vi "Actor Core.vi"(8 "error in":errorcluster, 11 "Lockin Processor in":refnum<class "Lockin Processor.lvclass">) -> (0 "error out":errorcluster, 3 "Actor out":refnum<class "Actor.lvclass">)   [LabVIEW 2016, in "Lockin Processor.lvclass"]
doc: "(<B>Filename</B>: Actor Framework.lvlib:Actor.lvclass:Actor Core.vi)\n\nReceives messages to the actor, reacts to them, and initiates any error handling that may shut the actor down.\n\nDescendant classes may override this VI to append parallel tasks for the actor to complete while it handles messages. Overrides use the Call Parent Method node."
uses:
  Lockin Processor.lvclass
  C:/github/LabActor/Template Module/Template Module.lvclass
  C:/Program Files/National Instruments/LabVIEW 2016/vi.lib/ActorFramework/Actor/Actor.lvclass
  <vilib>/ActorFramework/Actor/Actor.lvclass
  Lockin Processor Configuration.ctl
  Lockin Processor.lvclass/Lockin Processor.ctl
  Template Module/Template Module.lvclass/Template Module.ctl
  <vilib>/ActorFramework/Actor/Actor.lvclass/Actor.ctl
  <vilib>/ActorFramework/Message Enqueuer/Message Enqueuer.lvclass/Message Enqueuer.ctl
  NHMFL_Core/Libraries/Instruments/Results/File Path Result/File Path Result.lvclass
  C:/github/NHMFL_Core/Libraries/Instruments/Results/Acquired Result/Acquired Result.lvclass
  Process Object Messages/Process Result Msg/Process Result Msg.lvclass/Process Result Msg.ctl
  Template Module/Read stop event.vi
  <vilib>/ActorFramework/Message Enqueuer/Init from Existing Queue.vi
  <vilib>/ActorFramework/Message Enqueuer/Enqueue.vi
  Process Object Messages/Process Result Msg/Process Result Msg.lvclass
  C:/Program Files/National Instruments/LabVIEW 2016/vi.lib/ActorFramework/Message/Message.lvclass
  Lockin Processor Messages/Update Plot Msg/Update Plot Msg.lvclass
  <vilib>/ActorFramework/Message Priority Queue/Priority Enqueue.vi
  Process Object/Process Object.lvclass
  <vilib>/ActorFramework/Message Enqueuer/Message Enqueuer.lvclass
panel:
  out "Name":string
  in  "Re-process":bool
  out "XY Graph":cluster{dbl[], "Y":dbl[]}[](graph)
  in  "Input file":path
  in  "Configuration":T1={"Time constant"=0.0001, "Signal channels"=["V"], "Group"="p", "X channel"="Field", "Live update"=TRUE, "Phases"=[], "Harmonics"=[]} {"Phases" scale=-180.0..180.0; "Time constant" min=1e-06 max=1.0 scale=1e-06..0.01 scale format="%#_6p"}
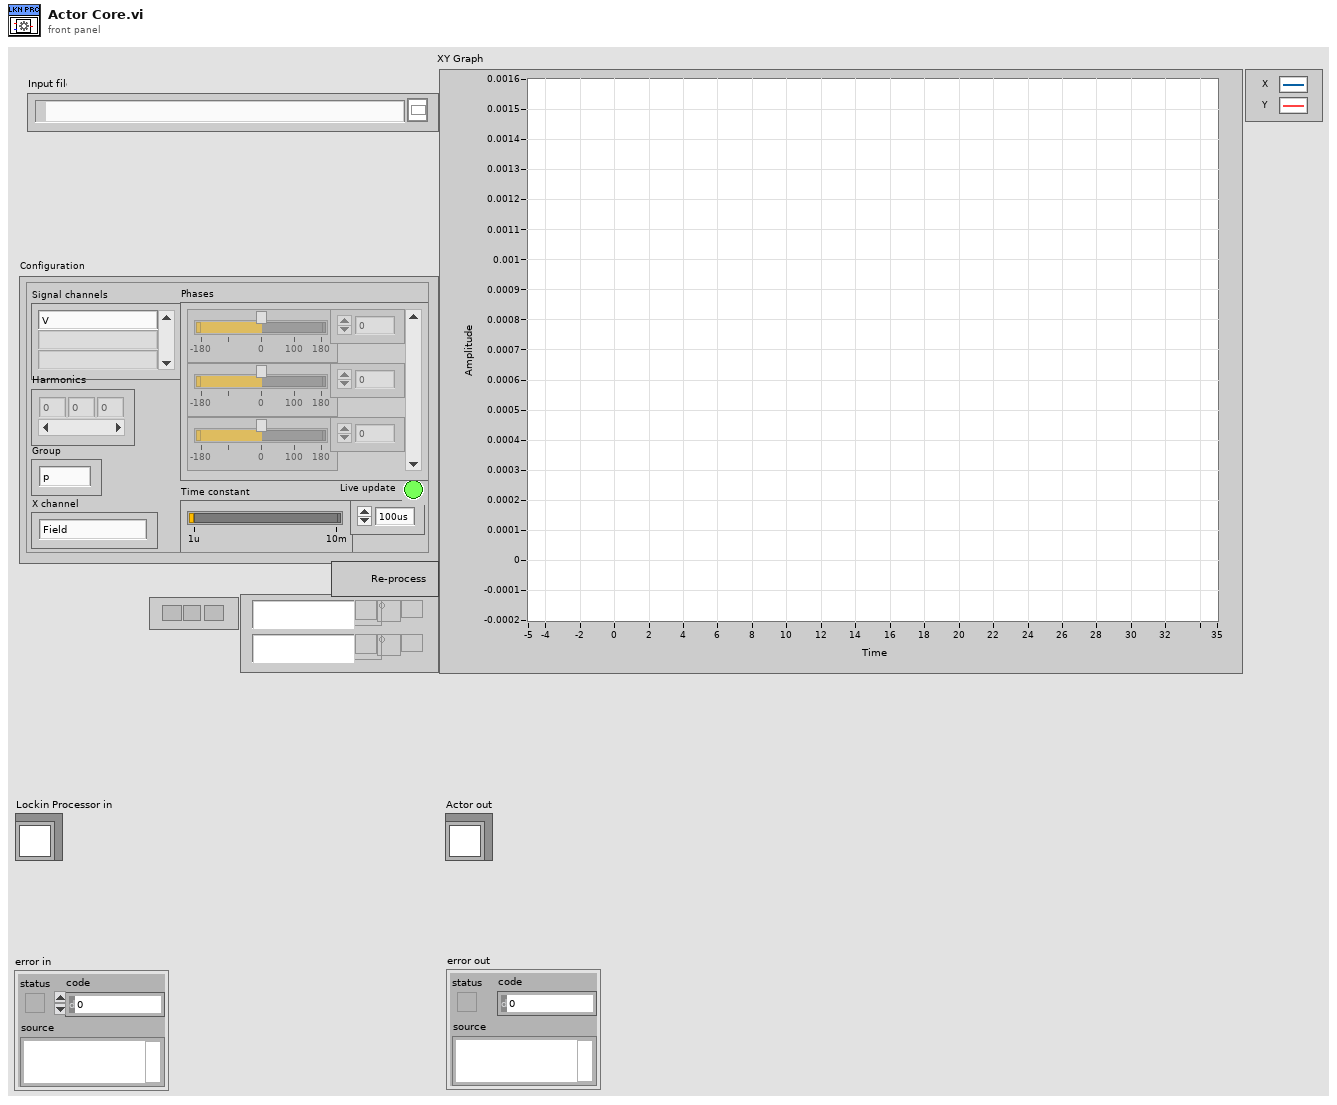
[diagram p1: front panel]
types:
  T1 = typedef "Lockin Processor Configuration.ctl" = cluster{"Time constant":dbl, "Signal channels":string[], "Group":string, "X channel":string, "Live update":bool, "Phases":dbl[], "Harmonics":i32[]}
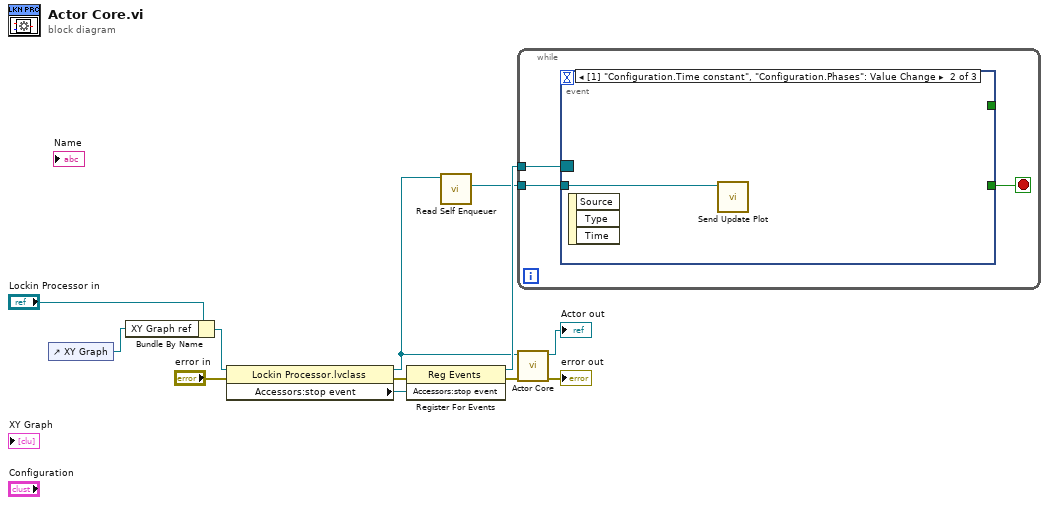
[diagram p0: block diagram]
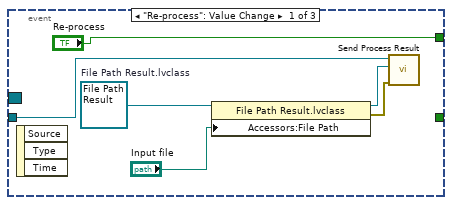
[diagram p2: hidden frame]
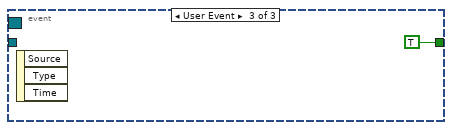
[diagram p3: hidden frame]
diagram:
  n1 = control-ref of="XY Graph"() -> (w1:refnum<vi>)
  n2 = Bundle By Name(cluster="Lockin Processor in", "XY Graph ref"=w1) -> (w2:refnum<class "Lockin Processor.lvclass">)
  n3 = property class="Lockin Processor.lvclass"(reference=w2, error in="error in") -> (reference out=w4:refnum<class "Lockin Processor.lvclass">, error out=w7:errorcluster, "Accessors:stop event"=w9:refnum<user-event>)
  n4 = register-events(error in=w7, w9) -> (reference out=w8:refnum<event-registration>, error out=w6:errorcluster)  [unwired: 1 in]
  n5 = call <vilib>:"Read Self Enqueuer.vi"("Actor"=w4) -> ("Self Enqueuer"=w3:refnum<class "Message Enqueuer.lvclass">)  [unwired: 10 in]
  n6 = while {
    tunnel: w8 -> [w15]
    tunnel: w3 -> [w13]
    stop <- w14 stop-if-true
    n7 = event shown="[1] \"Configuration.Time constant\", \"Configuration.Phases\": Value Change" {
      selector: w15 -> [_ _ _]
      dyn-events: _ -> [_ _ _]
      timeout: _ -> [_ _ _]
      tunnel: [_ _ TRUE] -> w14
      tunnel: w13 -> [w21 w22 _]
      tunnel: ["Re-process" _ _] -> _
      event "Re-process": Value Change {
        w20 = refnum<class "File Path Result.lvclass"> refnum  # File Path Result.lvclass
        n8 = event-data() -> ()  [unwired: 1 in, 3 out]
        n9 = property class="File Path Result.lvclass"(reference=w20, "Accessors:File Path"="Input file") -> (reference out=w19:refnum<class "File Path Result.lvclass">, error out=w18:errorcluster)  [unwired: 1 in]
        n10 = call "Send Process Result.vi"("error in (no error)"=w18, "Result in"=w19, "Message Enqueuer"=w21) -> ()  [unwired: 7 in, 2 out]
      }
      event Value Change {
        n11 = event-data() -> ()  [unwired: 1 in, 3 out]
        n12 = call "Send Update Plot.vi"("Message Enqueuer"=w22) -> ()  [unwired: 9 in, 2 out]
      }
      event User Event {
        n13 = event-data() -> ()  [unwired: 1 in, 3 out]
      }
    }
  }
  n14 = call-parent "Actor Core.vi"("error in"=w6, "Measure Object in"=w4) -> ("error out"=→"error out":errorcluster, "Actor out"=→"Actor out":refnum<class "Actor.lvclass">)  [unwired: 8 in]
